vi "Organize Scouting Data.vi"() -> ()   [LabVIEW 2015]
uses:
  <vilib>/Utility/sysdir.llb/System Directory Type.ctl
panel:
  in  "Sort By":u16(ring) items=["Team Number", "Rating", "Number of High Goals", "Number of Low Goals"]
  out "Array2":string[][](array[string])
  in  "array type (2D Dbl)":string[][](array[string])
  # "Team Number"
  # "Lift Gate"
  # "Teeter Totter"
  # "Moat"
  # "Rampart"
  # "Drawbridge"
  # "Sally Port"
  # "Rock Wall"
  # "Rough Terrain"
  # "Low Bar"
  # "Auto High Goal"
  # "Auto Low Goal"
  # "Scale"
  # "High Goals"
  # "Low Goal"
  # "Autonomous"
  # "Up to Defense"
  # "Rating"
  # "Comment"
  # "Team Number"
  # "Lift Gate"
  # "Teeter Totter"
  # "Moat"
  # "Rampart"
  # "Drawbridge"
  # "Sally Port"
  # "Rock Wall"
  # "Rough Terrain"
  # "Low Bar"
  # "Auto High Goal"
  # "Auto Low Goal"
  # "Scale"
  # "High Goals"
  # "Low Goal"
  # "Autonomous"
  # "Up to Defense"
  # "Rating"
  # "Comment"
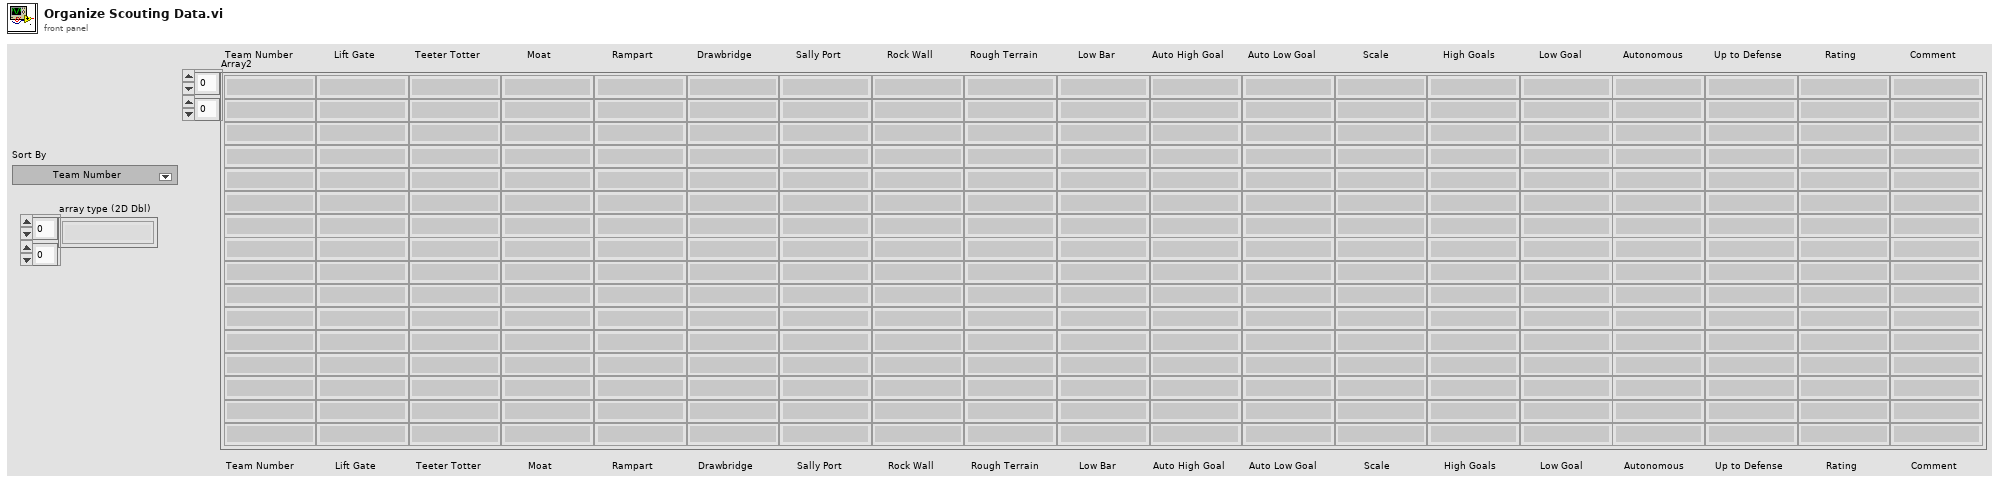
[diagram p1: front panel]
types:
  T1 = typedef "System Directory Type.ctl" = i32
  T2 = cluster{string, string, string, string, string, string, string, string, string, string, string, string, string, string, string, string, string, string, string}[]
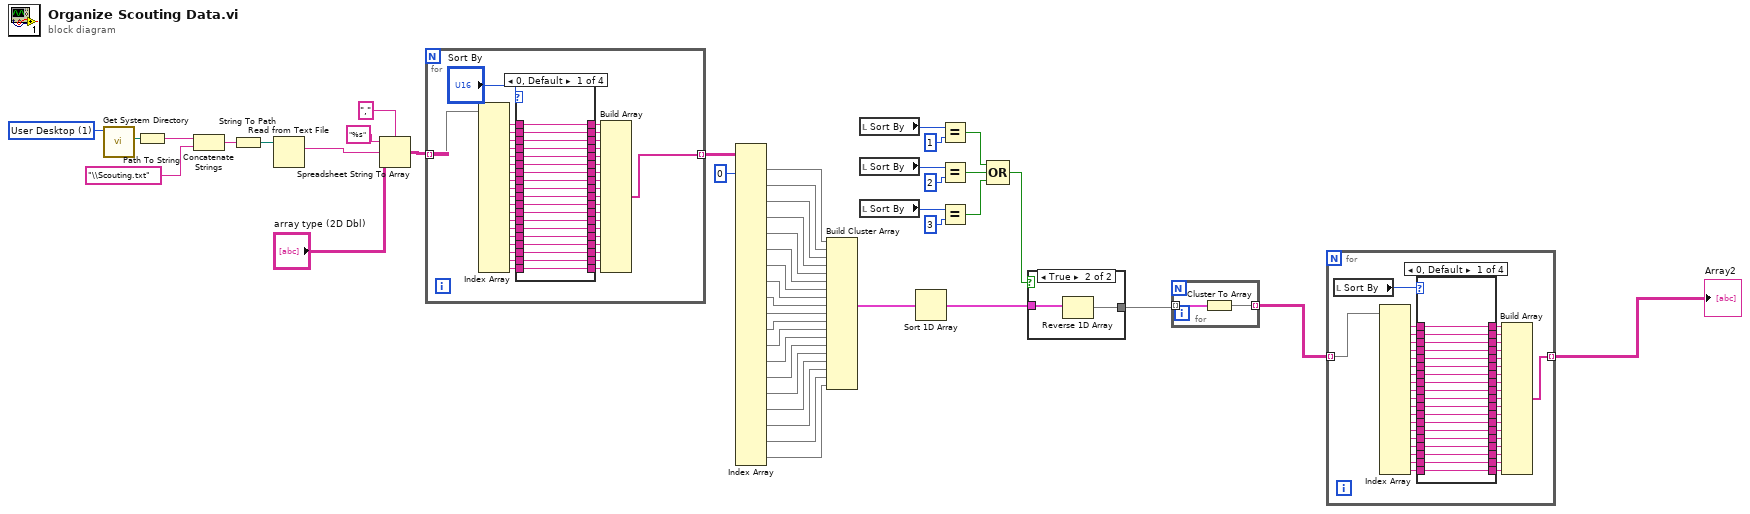
[diagram p0: block diagram]
diagram:
  w43 = T1 1 items=["User Home"=0, "User Desktop"=1, "User Documents"=2, "User Application Data"=3, "User Preferences"=4, "User Temporary"=5, "Public Documents"=6, "Public Application Data"=7, "Public Preferences"=8, "Public Cache"=13, "System Core Libraries"=9, "System Installed Libraries"=10, "Application Files"=11, "Boot Volume Root"=12] ("system directory type")
  n1 = call <vilib>:"Get System Directory.vi"("system directory type"=w43) -> ("system directory"=w44:path)  [unwired: 10 in]
  n2 = Path To String(path=w44) -> (string=w45:string)
  n3 = Concatenate Strings(w45, "\\Scouting.txt" ("string")) -> (w47:string)
  n4 = String To Path(string=w47) -> (path=w42:path)
  n5 = Read from Text File(file (use dialog)=w42) -> (text=w39:string)  [unwired: 3 in, 3 out]
  n6 = Spreadsheet String To Array(delimiter (Tab)=",", format string="%s", spreadsheet string=w39, array type (2D Dbl)="array type (2D Dbl)") -> (array=w17:string[][])
  n7 = for {
    tunnel: w17 -> [w88] mode=indexing
    tunnel: [w51] -> w16 mode=indexing
    n8 = Index Array(array=w88) -> (element #1=w86:string, element #2=w84:string, element #3=w83:string, element #4=w80:string, element #5=w78:string, element #6=w76:string, element #7=w74:string, element #8=w72:string, element #9=w70:string, element #10=w68:string, element #11=w66:string, element #12=w64:string, element #13=w62:string, element #14=w60:string, element #15=w58:string, element #16=w56:string, element #17=w54:string, element #18=w52:string, element #19=w48:string)  [unwired: 19 in]
    n9 = case shown="0, Default" "Sort By" {
      tunnel: [w107 w125 w145 w147] -> w87
      tunnel: w86 -> [w107 w126 w144 w148]
      tunnel: [w106 w124 w143 w164] -> w85
      tunnel: w84 -> [w106 w124 w143 w164]
      tunnel: [w105 w123 w142 w163] -> w82
      tunnel: w83 -> [w105 w123 w142 w163]
      tunnel: [w104 w122 w141 w162] -> w81
      tunnel: w80 -> [w104 w122 w141 w162]
      tunnel: [w103 w121 w140 w161] -> w79
      tunnel: w78 -> [w103 w121 w140 w161]
      tunnel: [w102 w120 w139 w160] -> w77
      tunnel: w76 -> [w102 w120 w139 w160]
      tunnel: [w101 w119 w138 w159] -> w75
      tunnel: w74 -> [w101 w119 w138 w159]
      tunnel: [w100 w118 w137 w158] -> w73
      tunnel: w72 -> [w100 w118 w137 w158]
      tunnel: [w99 w117 w136 w157] -> w71
      tunnel: w70 -> [w99 w117 w136 w157]
      tunnel: [w98 w116 w135 w156] -> w69
      tunnel: w68 -> [w98 w116 w135 w156]
      tunnel: [w97 w115 w134 w155] -> w67
      tunnel: w66 -> [w97 w115 w134 w155]
      tunnel: [w96 w114 w133 w154] -> w65
      tunnel: w64 -> [w96 w114 w133 w154]
      tunnel: [w95 w113 w132 w153] -> w63
      tunnel: w62 -> [w95 w113 w132 w153]
      tunnel: [w94 w112 w144 w146] -> w61
      tunnel: w60 -> [w94 w112 w145 w146]
      tunnel: [w93 w111 w131 w148] -> w59
      tunnel: w58 -> [w93 w111 w131 w147]
      tunnel: [w92 w110 w130 w152] -> w57
      tunnel: w56 -> [w92 w110 w130 w152]
      tunnel: [w91 w109 w129 w151] -> w55
      tunnel: w54 -> [w91 w109 w129 w151]
      tunnel: [w90 w126 w128 w150] -> w53
      tunnel: w52 -> [w90 w125 w128 w150]
      tunnel: [w89 w108 w127 w149] -> w49
      tunnel: w48 -> [w89 w108 w127 w149]
      frame 0, Default {
      }
      frame 1 {
      }
      frame 2 {
      }
      frame 3 {
      }
    }
    n10 = Build Array(w87, w85, w82, w81, w79, w77, w75, w73, w71, w69, w67, w65, w63, w61, w59, w57, w55, w53, w49) -> (w51:string[])
  }
  n11 = Index Array(array=w16, index (col) #1=0 ("disabled index (col)")) -> (element #1=w37:string[], element #2=w36:string[], element #3=w35:string[], element #4=w34:string[], element #5=w33:string[], element #6=w32:string[], element #7=w31:string[], element #8=w30:string[], element #9=w29:string[], element #10=w28:string[], element #11=w27:string[], element #12=w26:string[], element #13=w25:string[], element #14=w24:string[], element #15=w23:string[], element #16=w22:string[], element #17=w21:string[], element #18=w20:string[], element #19=w18:string[])  [unwired: 37 in]
  n12 = Build Cluster Array ("Index & Bundle Cluster Array")(w37, w36, w35, w34, w33, w32, w31, w30, w29, w28, w27, w26, w25, w24, w23, w22, w21, w20, w18) -> (w19:T2)
  n13 = local read "Sort By"() -> (w13:u16)
  n14 = local read "Sort By"() -> (w10:u16)
  n15 = local read "Sort By"() -> (w9:u16)
  n16 = Sort 1D Array(array=w19) -> (sorted array=w15:T2)
  n17 = Equal?(x=w13, y=u16 1) -> (x = y?=w7:bool)
  n18 = Equal?(x=w10, y=u16 2) -> (x = y?=w6:bool)
  n19 = Equal?(x=w9, y=u16 3) -> (x = y?=w5:bool)
  n20 = Compound Arithmetic op=OR(w7, w6, w5) -> (w4:bool)
  n21 = case shown="True" w4 {
    tunnel: w15 -> [w165 w167]
    tunnel: [w165 w166] -> w14
    frame False {
    }
    frame True {
      n22 = Reverse 1D Array(array=w167) -> (reversed array=w166:T2)
    }
  }
  n23 = for {
    tunnel: w14 -> [w168] mode=indexing
    tunnel: [w169] -> w3 mode=indexing
    n24 = Cluster To Array(cluster=w168) -> (array=w169:string[])
  }
  n25 = for {
    tunnel: w3 -> [w210] mode=indexing
    tunnel: [w173] -> w1 mode=indexing
    n26 = local read "Sort By"() -> (w170:u16)
    n27 = Index Array(array=w210) -> (element #1=w208:string, element #2=w206:string, element #3=w205:string, element #4=w202:string, element #5=w200:string, element #6=w198:string, element #7=w196:string, element #8=w194:string, element #9=w192:string, element #10=w190:string, element #11=w188:string, element #12=w186:string, element #13=w184:string, element #14=w182:string, element #15=w180:string, element #16=w178:string, element #17=w176:string, element #18=w174:string, element #19=w171:string)  [unwired: 19 in]
    n28 = case shown="0, Default" w170 {
      tunnel: [w229 w247 w267 w269] -> w209
      tunnel: w208 -> [w229 w248 w266 w270]
      tunnel: [w228 w246 w265 w286] -> w207
      tunnel: w206 -> [w228 w246 w265 w286]
      tunnel: [w227 w245 w264 w285] -> w204
      tunnel: w205 -> [w227 w245 w264 w285]
      tunnel: [w226 w244 w263 w284] -> w203
      tunnel: w202 -> [w226 w244 w263 w284]
      tunnel: [w225 w243 w262 w283] -> w201
      tunnel: w200 -> [w225 w243 w262 w283]
      tunnel: [w224 w242 w261 w282] -> w199
      tunnel: w198 -> [w224 w242 w261 w282]
      tunnel: [w223 w241 w260 w281] -> w197
      tunnel: w196 -> [w223 w241 w260 w281]
      tunnel: [w222 w240 w259 w280] -> w195
      tunnel: w194 -> [w222 w240 w259 w280]
      tunnel: [w221 w239 w258 w279] -> w193
      tunnel: w192 -> [w221 w239 w258 w279]
      tunnel: [w220 w238 w257 w278] -> w191
      tunnel: w190 -> [w220 w238 w257 w278]
      tunnel: [w219 w237 w256 w277] -> w189
      tunnel: w188 -> [w219 w237 w256 w277]
      tunnel: [w218 w236 w255 w276] -> w187
      tunnel: w186 -> [w218 w236 w255 w276]
      tunnel: [w217 w235 w254 w275] -> w185
      tunnel: w184 -> [w217 w235 w254 w275]
      tunnel: [w216 w234 w266 w268] -> w183
      tunnel: w182 -> [w216 w234 w267 w268]
      tunnel: [w215 w233 w253 w270] -> w181
      tunnel: w180 -> [w215 w233 w253 w269]
      tunnel: [w214 w232 w252 w274] -> w179
      tunnel: w178 -> [w214 w232 w252 w274]
      tunnel: [w213 w231 w251 w273] -> w177
      tunnel: w176 -> [w213 w231 w251 w273]
      tunnel: [w212 w248 w250 w272] -> w175
      tunnel: w174 -> [w212 w247 w250 w272]
      tunnel: [w211 w230 w249 w271] -> w172
      tunnel: w171 -> [w211 w230 w249 w271]
      frame 0, Default {
      }
      frame 1 {
      }
      frame 2 {
      }
      frame 3 {
      }
    }
    n29 = Build Array(w209, w207, w204, w203, w201, w199, w197, w195, w193, w191, w189, w187, w185, w183, w181, w179, w177, w175, w172) -> (w173:string[])
  }
  "Array2" <- w1
